vi "Probe (U128).vi"(9 "Data Valid":bool, 10 "input data":cluster{"high":u64, "low":u64}) -> (1 "Address":u64, 2 "Collected Data":cluster{"high":u64, "low":u64}[](array[cluster]))   [LabVIEW 2011]
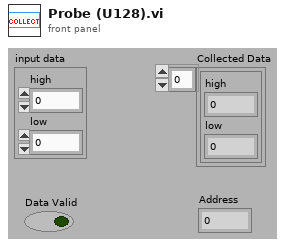
[diagram p1: front panel]
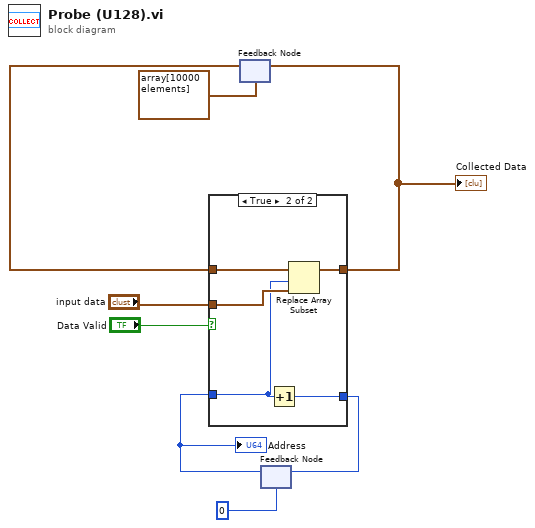
[diagram p0: block diagram]
diagram:
  n1 = feedback #1(cluster{"high":u64, "low":u64}[] array[10000 elements]) -> (w8:cluster{"high":u64, "low":u64}[])
  n2 = feedback #2(u64 0) -> (w1:u64)
  "Address" <- w1
  n3 = case shown="True" "Data Valid" {
    tunnel: "input data" -> [_ w15]
    tunnel: w8 -> [w10 w14]
    tunnel: [w10 w13] -> w3
    tunnel: w1 -> [w9 w11]
    tunnel: [w9 w12] -> w6
    frame False {
    }
    frame True {
      n4 = Increment(x=w11) -> (x+1=w12:u64)
      n5 = Replace Array Subset(array=w14, new element=w15, index=w11) -> (w13:cluster{"high":u64, "low":u64}[])
    }
  }
  "Collected Data" <- w3
  n6 = feedback-in #1(w3) -> ()
  n7 = feedback-in #2(w6) -> ()
